vi "TDMS Header Writer.vi"(8 "UserMetaData":T1 {"Amplifier Model" items=["Select a Model", "AM 1700", "BMA 200"]}, 11 "tdms file":refnum<k34>) -> (1 "Start Time hr/min":string, 2 "Date mm/dd/yy":string, 3 "tdms file out":refnum<k34>)   [LabVIEW 2014, in "Logging.lvlib"]
uses:
  Logging.lvlib
panel:
  out "error out":errorcluster
  # "Inputs"
  # "Outputs"
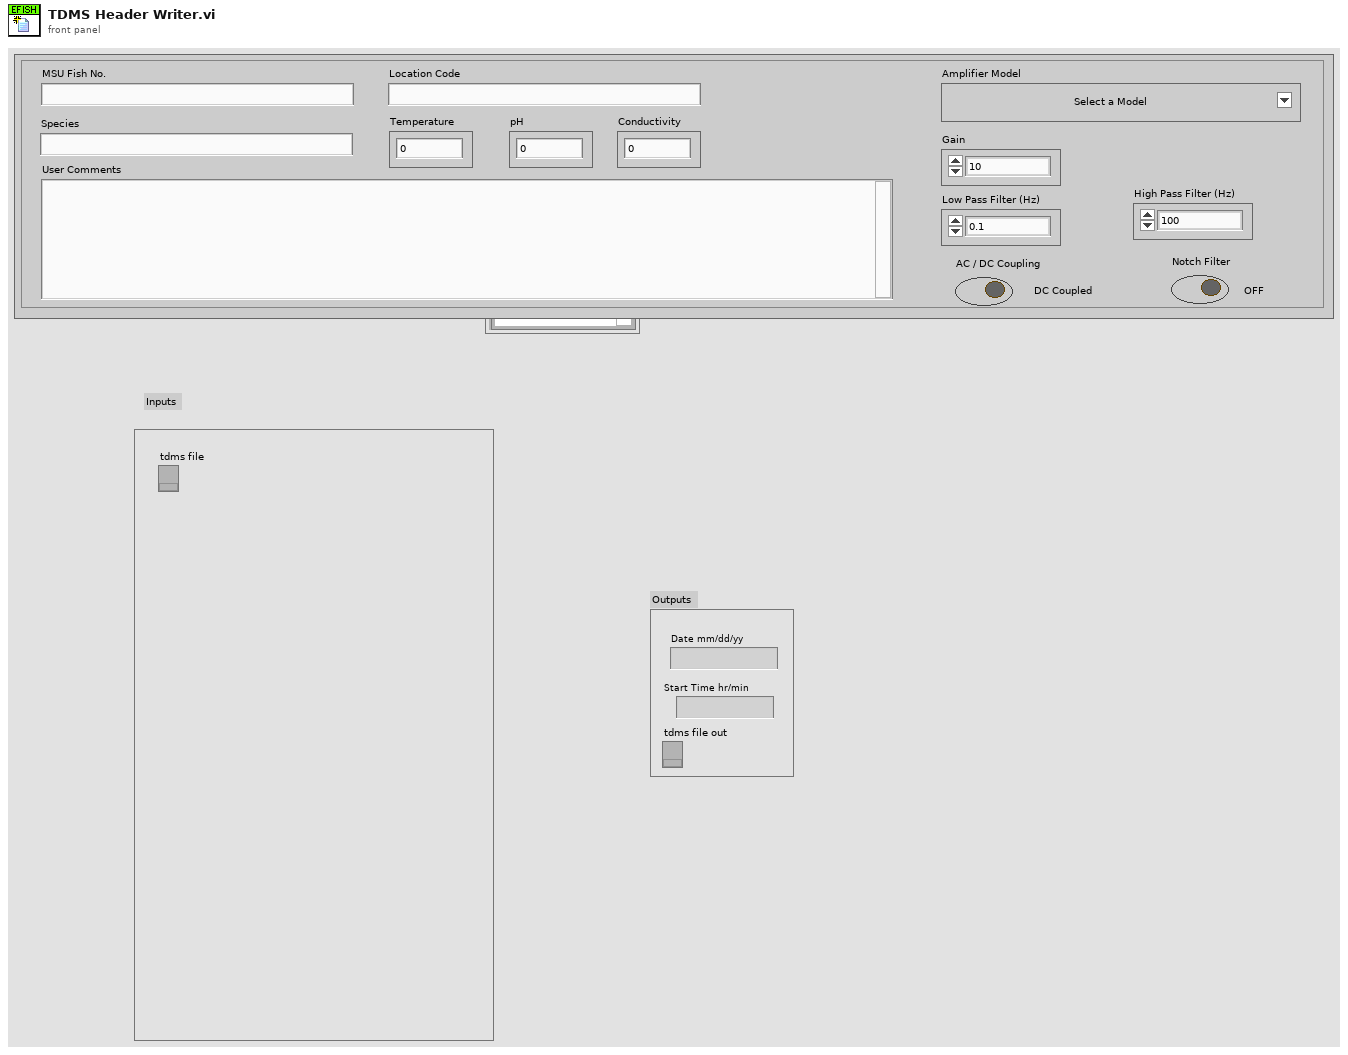
[diagram p1: front panel]
types:
  T1 = cluster{"MSU Fish No.":string, "Location Code":string, "Species":string, "Temperature":dbl, "pH":dbl, "Conductivity":dbl, "User Comments":string, "Amplifier Model":u16, "Gain":enum16{"10", "20", "50", "100", "200", "500", "1000", "2k", "5k", "10k", "20k", "50k"}, "Low Pass Filter (Hz)":enum16{"0.1", "1", "3", "10", "30", "100", "300"}, "High Pass Filter (Hz)":enum16{"100", "500", "1000", "3000", "5000", "10,000", "20,000", "30,000", "50,000"}, "AC / DC Coupling":bool, "Notch Filter":bool}
  T2 = enum16{"10", "20", "50", "100", "200", "500", "1000", "2k", "5k", "10k", "20k", "50k"}
  T3 = enum16{"0.1", "1", "3", "10", "30", "100", "300"}
  T4 = enum16{"100", "500", "1000", "3000", "5000", "10,000", "20,000", "30,000", "50,000"}
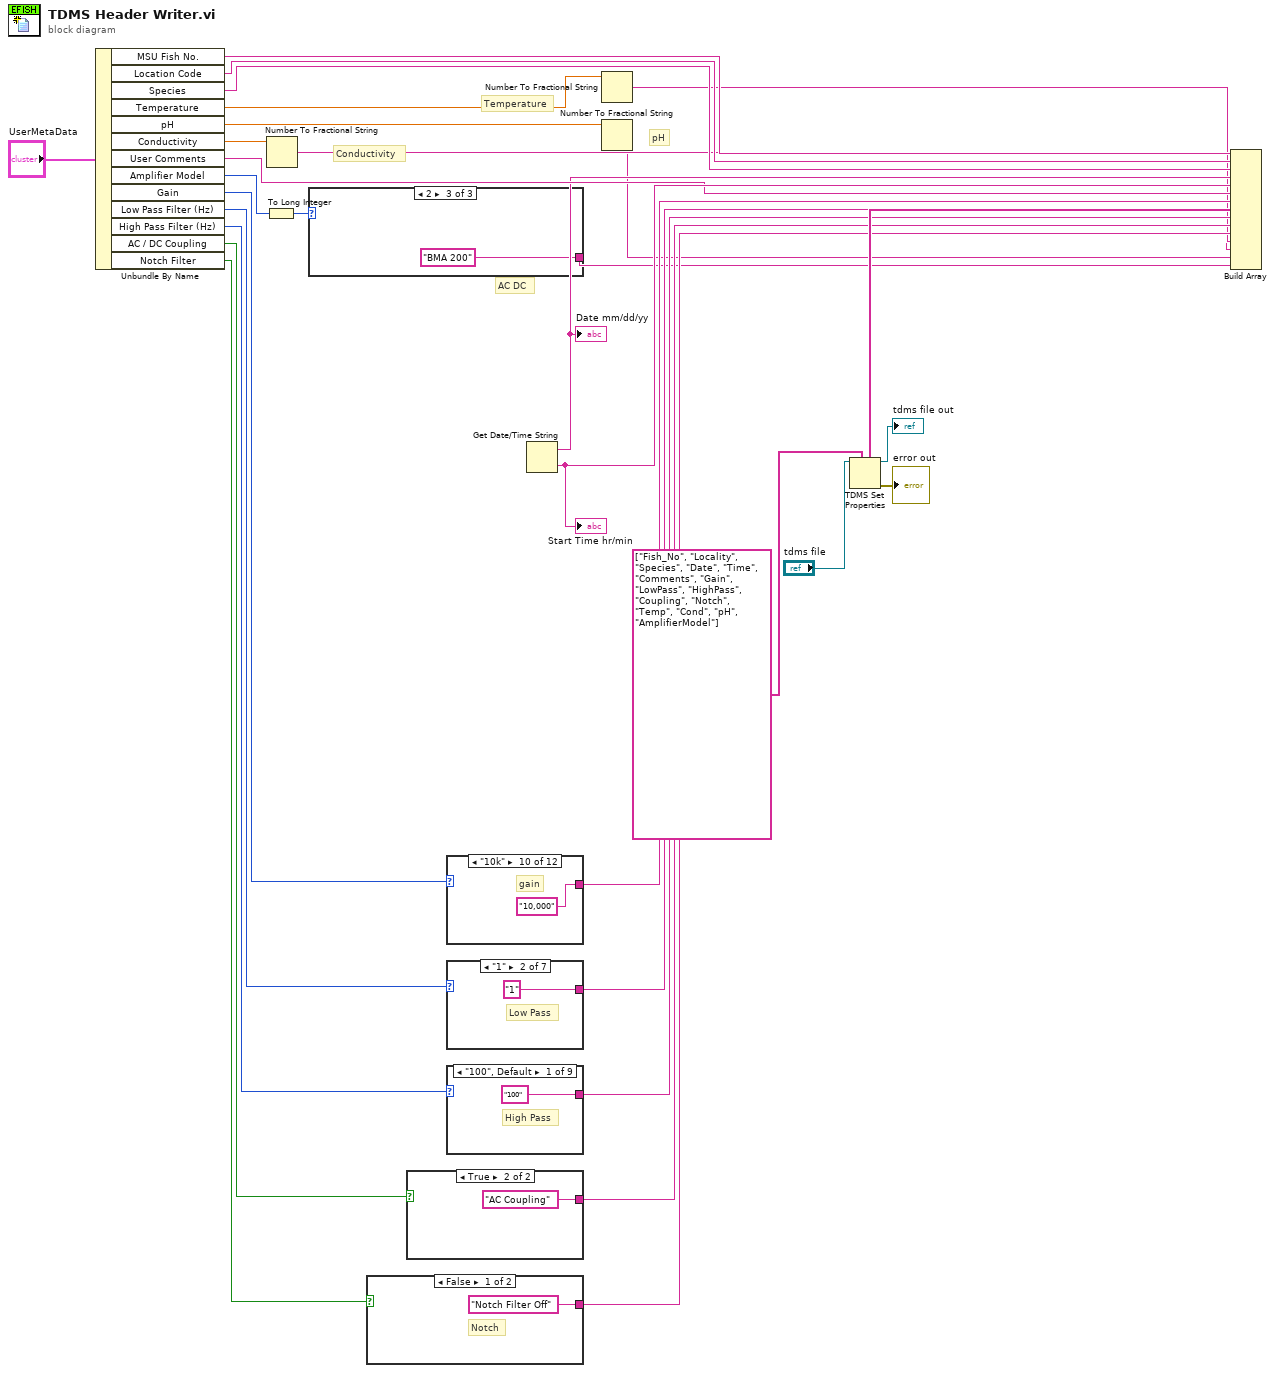
[diagram p0: block diagram]
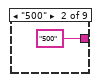
[diagram p2: hidden frame]
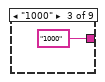
[diagram p3: hidden frame]
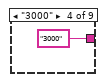
[diagram p4: hidden frame]
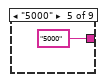
[diagram p5: hidden frame]
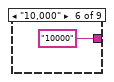
[diagram p6: hidden frame]
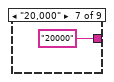
[diagram p7: hidden frame]
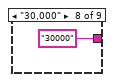
[diagram p8: hidden frame]
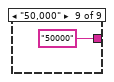
[diagram p9: hidden frame]
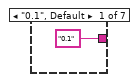
[diagram p10: hidden frame]
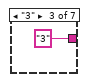
[diagram p11: hidden frame]
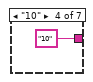
[diagram p12: hidden frame]
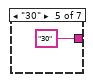
[diagram p13: hidden frame]
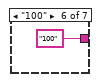
[diagram p14: hidden frame]
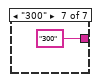
[diagram p15: hidden frame]
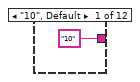
[diagram p16: hidden frame]
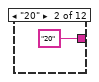
[diagram p17: hidden frame]
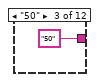
[diagram p18: hidden frame]
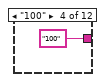
[diagram p19: hidden frame]
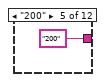
[diagram p20: hidden frame]
diagram:
  # "pH"
  # "Conductivity"
  # "Temperature"
  # "AC DC"
  n1 = Unbundle By Name("UserMetaData") -> ("MSU Fish No."=w18:string, "Location Code"=w17:string, "Species"=w16:string, "Temperature"=w15:dbl, "pH"=w13:dbl, "Conductivity"=w14:dbl, "User Comments"=w12:string, "Amplifier Model"=w11:u16, "Gain"=w10:T2, "Low Pass Filter (Hz)"=w9:T3, "High Pass Filter (Hz)"=w8:T4, "AC / DC Coupling"=w7:bool, "Notch Filter"=w6:bool)
  n2 = To Long Integer(number=w11) -> (32bit integer=w31:i32)
  n3 = Number To Fractional String(number=w14) -> (F-format string=w3:string)  [unwired: 3 in]
  n4 = case shown="2" w31 {
    tunnel: ["Amplifier Model,Not Identified" "AM 1700" "BMA 200"] -> w1
    frame 0, Default {
    }
    frame 1 {
    }
    frame 2 {
    }
  }
  n5 = case shown="False" w6 {
    tunnel: ["Notch Filter Off" "Notch Filter On"] -> w20
    frame False {
      # "Notch"
    }
    frame True {
    }
  }
  n6 = case shown="True" w7 {
    tunnel: ["DC Coupling" "AC Coupling"] -> w21
    frame False {
    }
    frame True {
    }
  }
  n7 = case shown="\"10k\"" w10 {
    tunnel: ["10" "20" "50" "100" "200" "500" "1000" "2000" "5000" "10,000" "20,000" "50,000"] -> w24
    frame "10", Default {
    }
    frame "20" {
    }
    frame "50" {
    }
    frame "100" {
    }
    frame "200" {
    }
    frame "500" {
    }
    frame "1000" {
    }
    frame "2k" {
    }
    frame "5k" {
    }
    frame "10k" {
      # "gain"
    }
    frame "20k" {
    }
    frame "50k" {
    }
  }
  n8 = case shown="\"1\"" w9 {
    tunnel: ["0.1" "1" "3" "10" "30" "100" "300"] -> w23
    frame "0.1", Default {
    }
    frame "1" {
      # "Low Pass"
    }
    frame "3" {
    }
    frame "10" {
    }
    frame "30" {
    }
    frame "100" {
    }
    frame "300" {
    }
  }
  n9 = case shown="\"100\", Default" w8 {
    tunnel: ["100" "500" "1000" "3000" "5000" "10000" "20000" "30000" "50000"] -> w22
    frame "100", Default {
      # "High Pass"
    }
    frame "500" {
    }
    frame "1000" {
    }
    frame "3000" {
    }
    frame "5000" {
    }
    frame "10,000" {
    }
    frame "20,000" {
    }
    frame "30,000" {
    }
    frame "50,000" {
    }
  }
  n10 = Get Date/Time String() -> (date string=w5:string, time string=w25:string)  [unwired: 3 in]
  "Date mm/dd/yy" <- w5
  "Start Time hr/min" <- w25
  n11 = Number To Fractional String(number=w15) -> (F-format string=w4:string)  [unwired: 3 in]
  n12 = Number To Fractional String(number=w13) -> (F-format string=w2:string)  [unwired: 3 in]
  n13 = Build Array(w18, w17, w16, w5, w25, w12, w24, w23, w22, w21, w20, w4, w3, w2, w1) -> (w29:string[])
  n14 = TDMS Set Properties(5:w29, 7:string[] ["Fish_No", "Locality", "Species", "Date", "Time", "Comments", "Gain", "LowPass", "HighPass", "Coupling", "Notch", "Temp", "Cond", "pH", "AmplifierModel"] ("property names"), 11:"tdms file") -> (0:→"error out":errorcluster, 3:→"tdms file out":refnum<k34>)  [unwired: 3 in, 2 out]
